vi "Rotate FGV.vi"(7 "State":T1, 8 "error in":errorcluster, 10 "Clockwise?":bool, 11 "Degrees Rotation":dbl format="%#_13g") -> (0 "error out":errorcluster, 1 "Complete?":bool, 2 "Right Setpoint":dbl, 3 "Left Setpoint":dbl)   [LabVIEW 2016]
doc: "Rotate source code FGV; calculates whether or not a rotation has completed based on difference in ticks between the left wheel and the right wheel."
uses:
  Rotate States.ctl
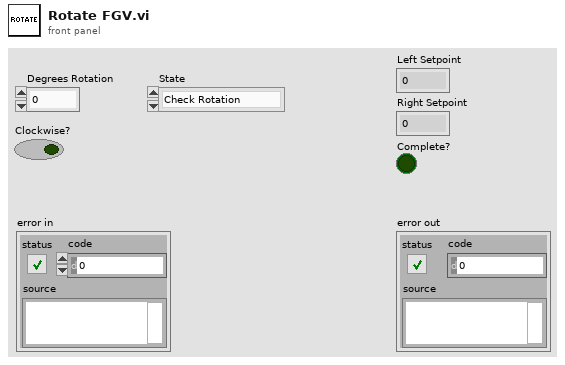
[diagram p1: front panel]
types:
  T1 = typedef "Rotate States.ctl" = enum16{"Check Rotation", "Initialize Rotation"}
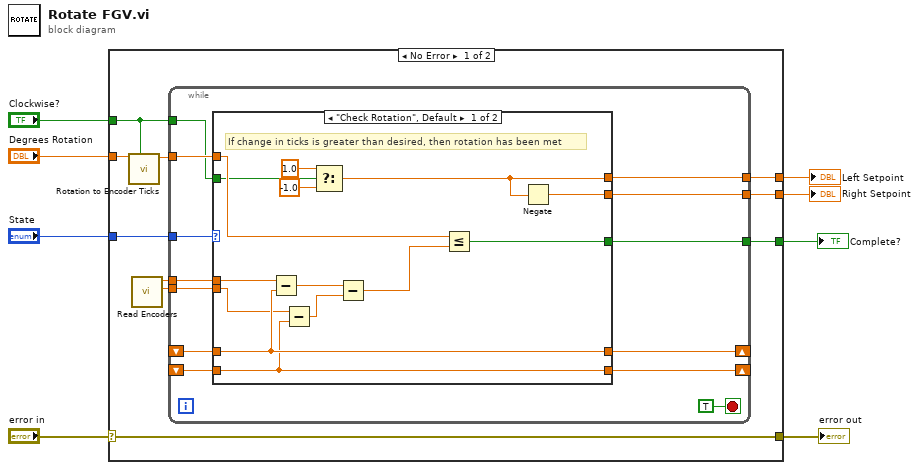
[diagram p0: block diagram]
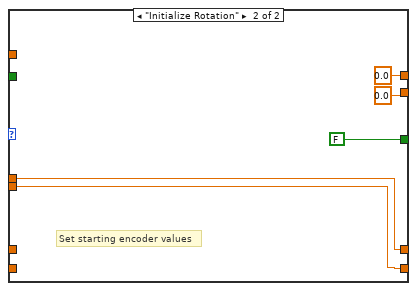
[diagram p2: hidden frame]
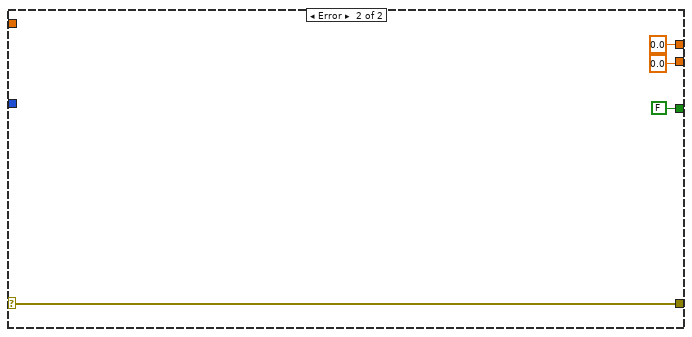
[diagram p3: hidden frame]
diagram:
  n1 = case shown="No Error" "error in" {
    selector: "error in" -> [w14 w54]
    tunnel: "State" -> [w18 _]
    tunnel: "Degrees Rotation" -> [w13 _]
    tunnel: [w15 FALSE] -> w6
    tunnel: [w14 w54] -> w4
    tunnel: "Clockwise?" -> [w11 _]
    tunnel: [w10 0.0 ("f")] -> w2
    tunnel: [w9 0.0] -> w1
    frame No Error {
      n2 = call "Rotation to Encoder Ticks.vi"("Clockwise?"=w11, "Degrees"=w13) -> ("Difference in Ticks"=w12:dbl)  [unwired: 9 in]
      n3 = call "Read Encoders.vi"() -> ("Right Encoder"=w16:dbl, "Left Encoder"=w17:dbl)  [unwired: 10 in]
      n4 = while {
        tunnel: w18 -> [w30]
        shift-right: [w29] -> _
        shift-left: _ -> [w27]
        shift-right: [w28] -> _
        shift-left: _ -> [w26]
        tunnel: w17 -> [w25]
        tunnel: w16 -> [w24]
        tunnel: w12 -> [w23]
        tunnel: [w22] -> w15
        tunnel: w11 -> [w21]
        tunnel: [w20] -> w10
        tunnel: [w19] -> w9
        stop <- TRUE ("stop") stop-if-true
        n5 = case shown="\"Check Rotation\", Default" w30 {
          tunnel: [w44 w50] -> w29
          tunnel: [w42 w49] -> w28
          tunnel: w27 -> [w44 _]
          tunnel: w26 -> [w42 _]
          tunnel: w25 -> [w45 w50]
          tunnel: w24 -> [w43 w49]
          tunnel: w23 -> [w38 _]
          tunnel: [w37 FALSE] -> w22
          tunnel: w21 -> [w36 _]
          tunnel: [w33 0.0 ("f")] -> w20
          tunnel: [w32 0.0] -> w19
          frame "Check Rotation", Default {
            # "If change in ticks is greater than desired, then rotation has been met"
            n6 = Subtract(x=w45, y=w44) -> (x-y=w41:dbl)
            n7 = Subtract(x=w43, y=w42) -> (x-y=w40:dbl)
            n8 = Select(t=1.0, s=w36, f=-1.0) -> (s? t:f=w33:dbl)
            n9 = Subtract(x=w41, y=w40) -> (x-y=w39:dbl)
            n10 = Less Or Equal?(x=w38, y=w39) -> (x <= y?=w37:bool)
            n11 = Negate(x=w33) -> (-x=w32:dbl)
          }
          frame "Initialize Rotation" {
            # "Set starting encoder values"
          }
        }
      }
    }
    frame Error {
    }
  }
  "Complete?" <- w6
  "error out" <- w4
  "Left Setpoint" <- w2
  "Right Setpoint" <- w1
